vi "PicoScope3000aExampleEts.vi"() -> ()   [LabVIEW 2010]
uses:
  shared/PicoBuffers.ctl
  shared/Buffer and Transfer Settings.ctl
  shared/Acquisition Settings.ctl
  PicoScope3000aLib/PicoScope3000aAnalogChannelSettings.ctl
panel:
  out "Properties Panel":T1 {"Max Total Capture Time Available (sec)" format="%.3p"; "Sample Frequency" format="%.3p"; "Sample Rate" format="%.3p"; "Max Samples Available" format="%.3p"; "Total Capture Time (sec)" format="%.3p"}
  out "EtsTimeValues":i64[](array[numeric])
  in  "etsInterleave":i16=40
  in  "etsCycles":i16=200
  out "Max etsInterleave":i16
  out "Max etsCycles":i16
  in  "Trigger Settings":T2={"Trigger Enabled"=TRUE, "Trigger Source"=enum."Channel A", "Trigger Threshold (volts)"=0.0, "Trigger Direction"=2, "Trigger Delay (samples)"=0, "Auto Trigger Time (ms)"=1000} {"Trigger Direction" items=["Above", "Below", "Rising", "Falling", "Rising or Falling"]}
  in  "ETS Mode":u32(ring)=1 items=["PS3000A_ETS_OFF", "PS3000A_ETS_FAST", "PS3000A_ETS_SLOW"]
  in  "Channel A Settings":T3={"Enabled"=TRUE, "Coupling"=1, "Range"=6, "Analogue Offset"=0.0, "Bandwidth Limit"=0} {"Bandwidth Limit" items=["Full", "20MHz"]; "Range" items=["10 mV", "20 mV", "50 mV", "100 mV", "200 mV", "500 mV", "1 V", "2 V", "5 V", "10 V", "20 V", "50 V ", "100 V"]; "Coupling" items=["AC", "DC"]}
  out "overflow":i16 format="%010b"
  in  "Apply Settings":bool
  out "USB 3.0 device on non-USB 3.0 Port":bool=TRUE
  out "USB Powered":bool=TRUE
  out "Device Info":T4={"Driver Version"="0", "USB Version"="0", "Hardware"="0", "Variant"="0", "Batch and Serial"="0", "Cal Date"="0", "Kernel Version"="0", "Digital HW Version"="0", "Analogue HW Version"="0", "MSO"=FALSE, "Number of channels"=0}
  out "error out":errorcluster
  in  "Data file":path=path "PicoScope3000aExampleETS ChA Data"
  in  "Buffer and Transfer Settings":T5={"startIndex"=0, "Samples"=1000, "Down Sample Ratio"=1, "Down-Sample Mode"=0} {"Down-Sample Mode" items=["RAW none"=2147483648, "None"=0, "Aggregate"=1, "Decimate"=2, "Average"=4]; "Down Sample Ratio" step=1; "Samples" format="%_6p"}
  in  "Acquisition Settings":T6={"preTriggerSamples"=0, "postTriggerSamples"=1000, "timebase"=0} {"postTriggerSamples" format="%_6p"; "preTriggerSamples" format="%_6p"}
  in  "stop":bool
  out "Channel A":cluster{i32, sgl, "Data":dbl[]}(graph)
  in  "Serial Number":string
  in  "Use Serial Number":bool
  in  "error in (no error)":errorcluster
  # "Bit 0 = ChA"
  # "ETS mode on channel A only"
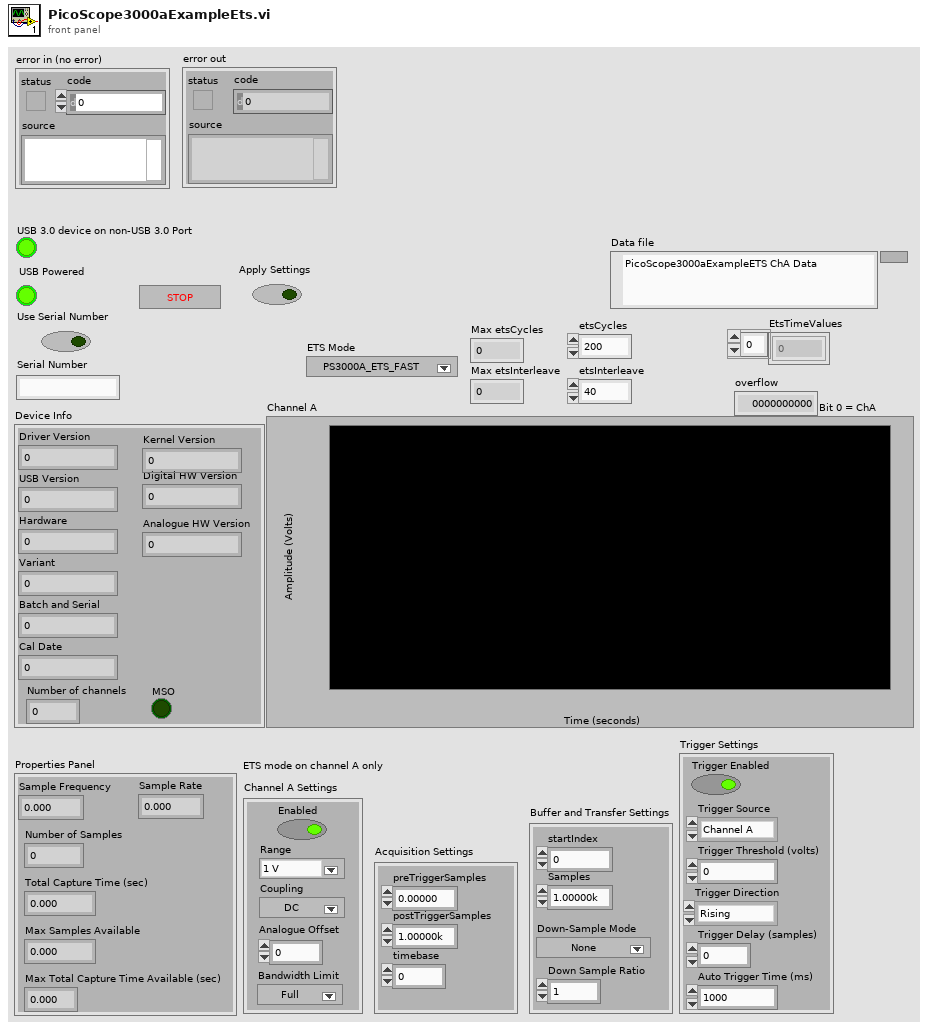
[diagram p1: front panel]
types:
  T1 = cluster{"Sample Frequency":sgl, "Sample Rate":sgl, "Max Samples Available":i32, "Number of Samples":u32, "Total Capture Time (sec) ":sgl, "Max Total Capture Time Available (sec)":sgl}
  T2 = cluster{"Trigger Enabled":bool, "Trigger Source":enum32{"Channel A", "Channel B", "Channel C", "Channel D", "Ext."}, "Trigger Threshold (volts)":dbl, "Trigger Direction":u32, "Trigger Delay (samples)":u32, "Auto Trigger Time (ms)":i16}
  T3 = typedef "PicoScope3000aAnalogChannelSettings.ctl" = cluster{"Enabled":bool, "Coupling":u32, "Range":u32, "Analogue Offset":sgl, "Bandwidth Limit":u32}
  T4 = cluster{"Driver Version":string, "USB Version":string, "Hardware":string, "Variant":string, "Batch and Serial":string, "Cal Date":string, "Kernel Version":string, "Digital HW Version":string, "Analogue HW Version":string, "MSO":bool, "Number of channels":i16}
  T5 = typedef "Buffer and Transfer Settings.ctl" = cluster{"startIndex":u64, "Samples":u64, "Down Sample Ratio":u64, "Down-Sample Mode":u32}
  T6 = typedef "Acquisition Settings.ctl" = cluster{"preTriggerSamples":u64, "postTriggerSamples":u64, "timebase":u32}
  T7 = typedef "PicoBuffers.ctl" = cluster{"Max Buffer Pointers":u64[][][], "Min Buffer Pointers":u64[][][], "StreamingDataInfo":cluster{"Channel":u32, "Down-Sample Mode":u32, "PICO_DATA_TYPE":enum32{"PICO_INT8_T", "PICO_INT16_T", "PICO_INT32_T", "PICO_UINT32_T", "PICO_INT64_T", ""}, "Samples":i32, "bufferIndex":u64, "startIndex":i32, "overflow":i16}[][]}
  T8 = enum16{"open", "open or create", "create or replace", "create", "open (read-only)"}
  T9 = cluster{"Channel A Buffer":i16[], "Channel B Buffer":i16[], "Channel C Buffer":i16[], "Channel D Buffer":i16[], "Channel E Buffer":i16[], "Channel F Buffer":i16[], "Channel G Buffer":i16[], "Channel H Buffer":i16[], "Port 0 Buffer":i16[], "Port 1 Buffer":i16[]}[]
  T10 = cluster{"Channel A Buffer":i16[], "Channel B Buffer":i16[], "Channel C Buffer":i16[], "Channel D Buffer":i16[], "Channel E Buffer":i16[], "Channel F Buffer":i16[], "Channel G Buffer":i16[], "Channel H Buffer":i16[], "Port 0 Buffer":i16[], "Port 1 Buffer":i16[]}
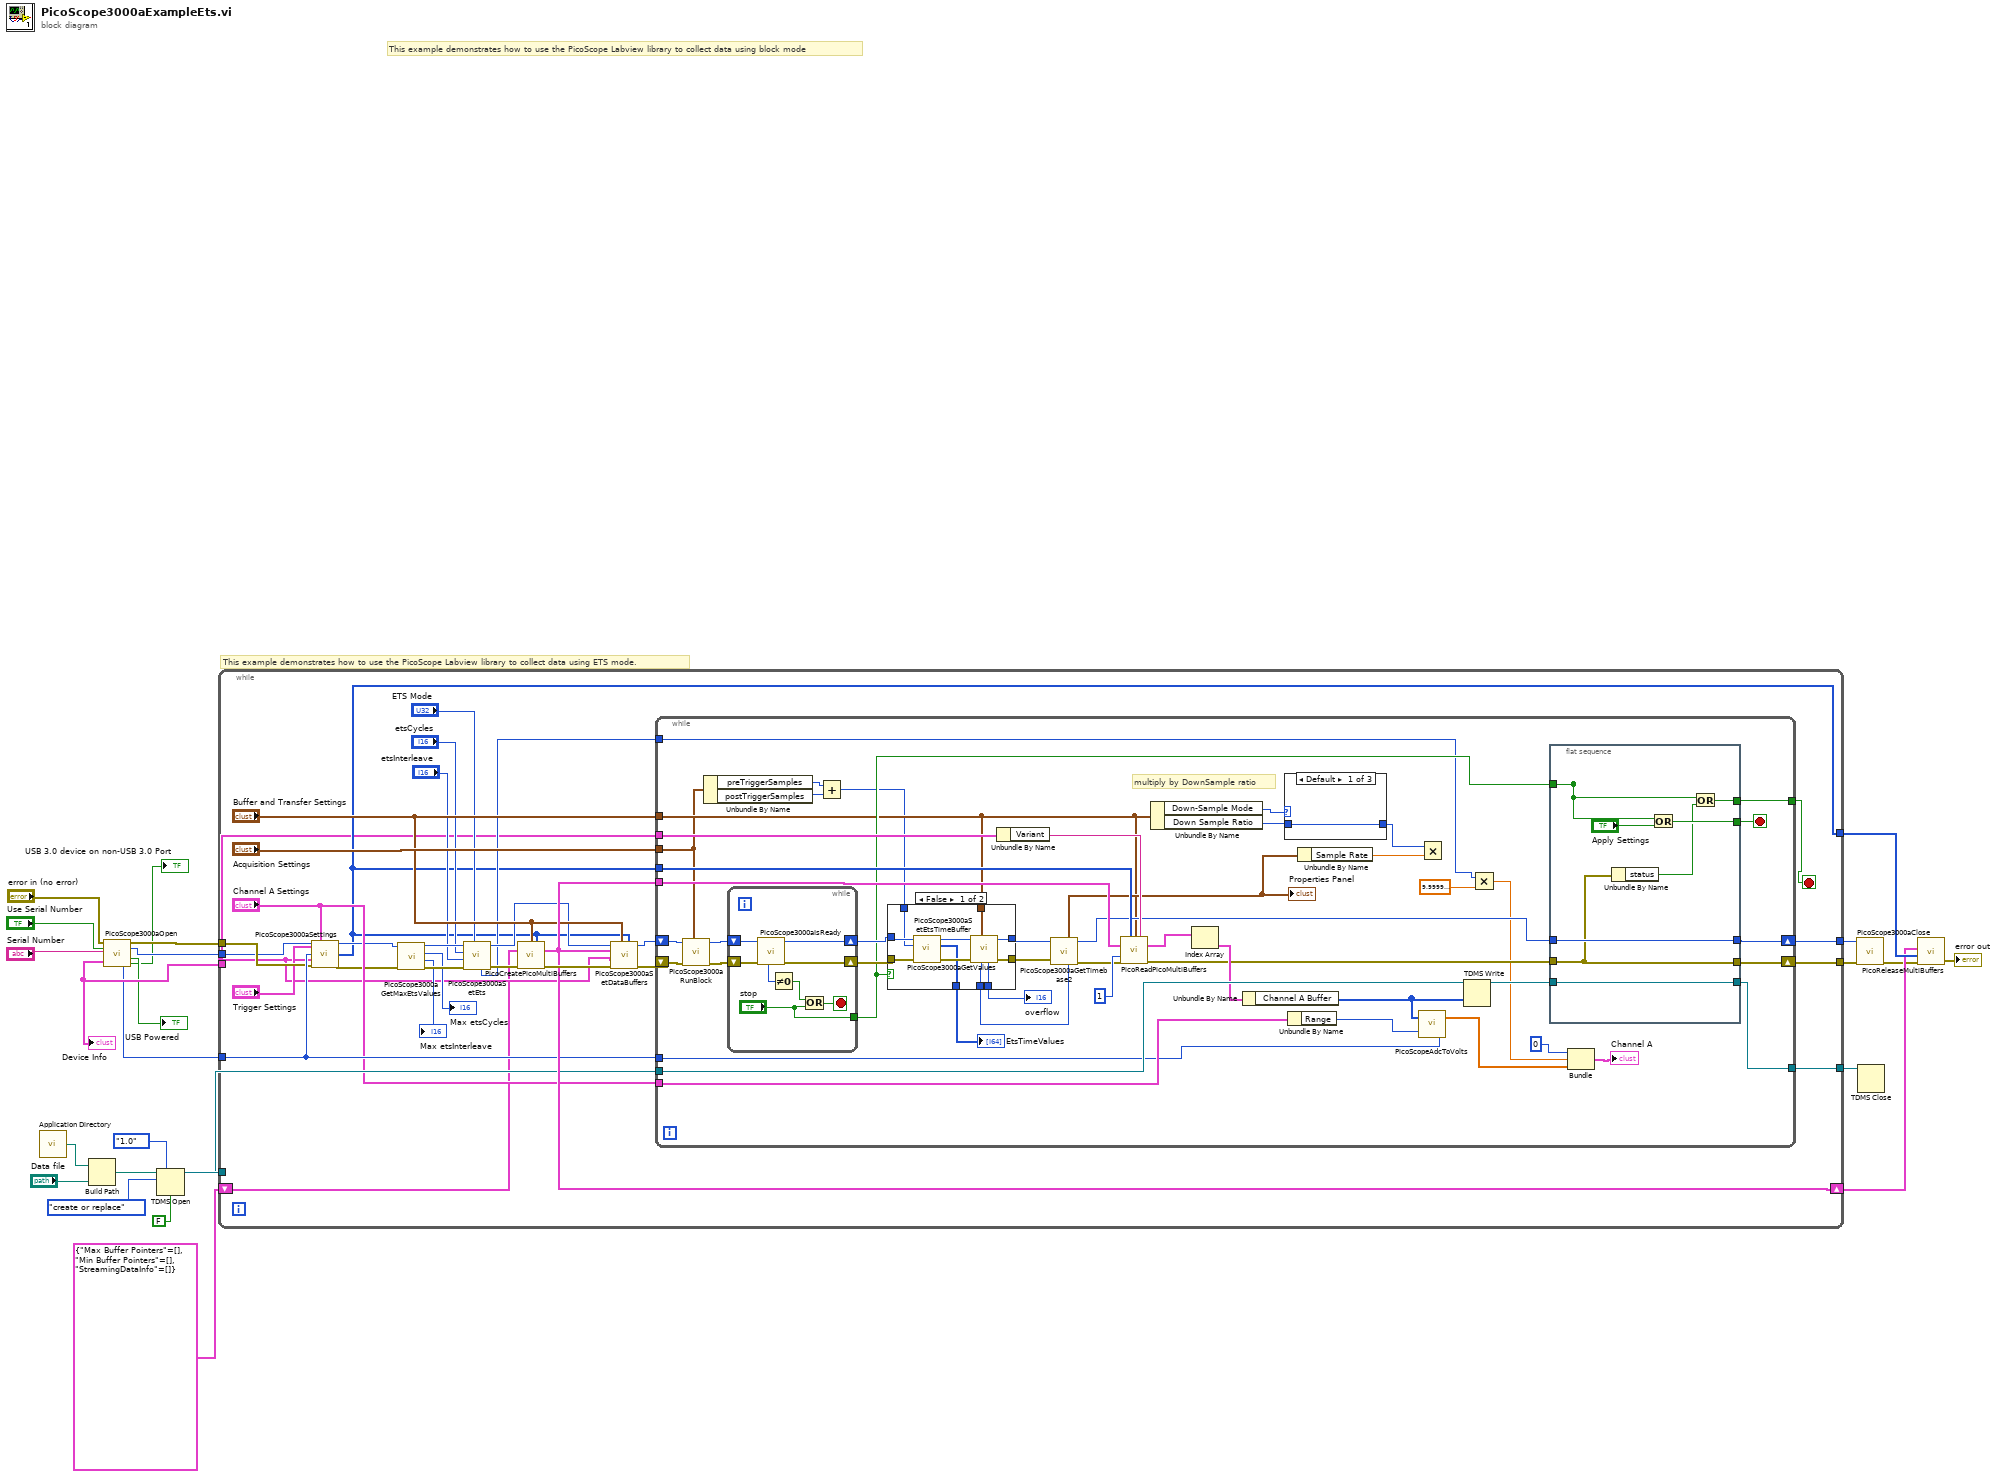
[diagram p0: block diagram]
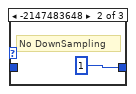
[diagram p3: hidden frame]
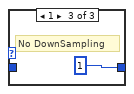
[diagram p4: hidden frame]
diagram:
  # "This example demonstrates how to use the PicoScope Labview library to collect data using ETS mode."
  # "This example demonstrates how to use the PicoScope Labview library to collect data using block mode"
  n1 = call <vilib>:"Application Directory.vi"() -> ("Application Directory"=w16:path)
  n2 = Build Path(base path=w16, name or relative path="Data file") -> (appended path=w17:path)
  n3 = call "PicoScope3000aOpen.vi"("error in (no error)"="error in (no error)", "Serial Number"="Serial Number", "Use Serial number"="Use Serial Number") -> ("error out"=w7:errorcluster, "handle"=w24:i16, "USB Powered"=→"USB Powered":bool, "Device Info"=w9:T4, "Max ADC value"=w5:i16, "USB 3.0 device on non-USB 3.0 Port"=→"USB 3.0 device on non-USB 3.0 Port":bool)  [unwired: 6 in, 1 out]
  "Device Info" <- w9
  n4 = TDMS Open(6:FALSE ("disable buffering? (T)"), 7:enum16{"1.0", "2.0"}."1.0" ("file format version (2.0)"), 10:T8."create or replace" ("operation (0:open)"), 11:w17) -> (3:w14:refnum<k34>)  [unwired: 2 in, 1 out]
  n5 = while {
    tunnel: w24 -> [w30]
    tunnel: w5 -> [w44]
    tunnel: [w28] -> w23
    tunnel: [w50] -> w15
    tunnel: w14 -> [w53]
    tunnel: w9 -> [w26]
    tunnel: w7 -> [w31]
    tunnel: [w51] -> w3
    tunnel: [w48] -> w6
    shift-right: [w54] -> w22
    shift-left: T7 {"Max Buffer Pointers"=[], "Min Buffer Pointers"=[], "StreamingDataInfo"=[]} ("Data Pointers") -> [w25]
    stop <- w49 stop-if-true
    n6 = call "PicoScope3000aSettings.vi"("handle in"=w30, "Channel A Settings"="Channel A Settings", "Trigger Settings"="Trigger Settings", "Max_adc"=w44, "Device Info"=w26, "error in"=w31) -> ("handle out"=w29:i16, "Enabled Array"=w28:i16[], "error out"=w32:errorcluster)  [unwired: 7 in]
    n7 = call "PicoScope3000aGetMaxEtsValues.vi"("error in (no error)"=w32, "handle in"=w29) -> ("error out"=w42:errorcluster, "Max etsInterleave"=→"Max etsInterleave":i16, "Max etsCycles"=→"Max etsCycles":i16, "handle out"=w39:i16)  [unwired: 6 in]
    n8 = call "PicoScope3000aSetEts.vi"("ETS Mode"="ETS Mode", "error in (no error)"=w42, "etsInterleave"="etsInterleave", "etsCycles"="etsCycles", "handle in"=w39) -> ("error out"=w41:errorcluster, "handle out"=w40:i16, "sampleTimePicoseconds"=w38:i32)  [unwired: 4 in]
    n9 = call "PicoCreatePicoMultiBuffers.vi"("Buffer and Transfer Settings"="Buffer and Transfer Settings", "enabled array"=w28, "Data Pointers In"=w25, "error in (no error)"=w41) -> ("Data Pointers"=w54:T7, "error out"=w55:errorcluster)  [unwired: 10 in]
    n10 = call "PicoScope3000aSetDataBuffers.vi"("enabled array"=w28, "Buffer and Transfer Settings"="Buffer and Transfer Settings", "error in (no error)"=w55, "Device Info"=w26, "Data Pointers In"=w54, "handle in"=w40) -> ("error out"=w47:errorcluster, "handle out"=w46:i16)  [unwired: 4 in]
    n11 = while {
      tunnel: w54 -> [w104]
      tunnel: "Buffer and Transfer Settings" -> [w66]
      tunnel: w28 -> [w96]
      tunnel: "Channel A Settings" -> [w95]
      tunnel: "Acquisition Settings" -> [w59]
      tunnel: w44 -> [w94]
      tunnel: w26 -> [w91]
      tunnel: [w81] -> w49
      shift-right: [w85] -> w51
      shift-left: w47 -> [w75]
      shift-right: [w79] -> w48
      shift-left: w46 -> [w76]
      tunnel: w53 -> [w103]
      tunnel: [w83] -> w50
      tunnel: w38 -> [w63]
      stop <- w80 stop-if-true
      # "multiply by DownSample ratio"
      n12 = call "PicoScope3000aRunBlock.vi"("Acquisition Settings"=w59, "error in (no error)"=w75, "handle in"=w76) -> ("error out"=w98:errorcluster, "handle out"=w97:i16)  [unwired: 5 in, 2 out]
      n13 = Unbundle By Name(w59) -> ("preTriggerSamples"=w58:u64, "postTriggerSamples"=w57:u64)
      n14 = while {
        shift-right: [w132] -> w77
        shift-left: w98 -> [w133]
        shift-right: [w131] -> w78
        shift-left: w97 -> [w130]
        tunnel: ["stop"] -> w74
        stop <- w127 stop-if-true
        n15 = call "PicoScope3000aIsReady.vi"("error in (no error)"=w133, "handle in"=w130) -> ("error out"=w132:errorcluster, "handle out"=w131:i16, "ready"=w129:i16)  [unwired: 7 in]
        n16 = Not Equal To 0?(x=w129) -> (x != 0?=w128:bool)
        n17 = Or(x=w128, y="stop") -> (x .or. y?=w127:bool)
      }
      n18 = Add(x=w58, y=w57) -> (x+y=w56:u64)
      n19 = case shown="False" w74 {
        tunnel: w77 -> [w110 w116]
        tunnel: w78 -> [w107 w117]
        tunnel: [w115 w117] -> w69
        tunnel: [w114 w116] -> w70
        tunnel: w66 -> [w113 _]
        tunnel: [w112 _] -> w73
        tunnel: [w111 _] -> w72
        tunnel: [w106 _] -> w62
        tunnel: w56 -> [w105 _]
        frame False {
          n20 = call "PicoScope3000aSetEtsTimeBuffer.vi"("error in (no error)"=w110, "bufferLth"=w105, "handle in"=w107) -> ("error out"=w109:errorcluster, "EtsTimeValues"=w106:i64[], "handle out"=w108:i16)  [unwired: 6 in]
          n21 = call "PicoScope3000aGetValues.vi"("Buffer and Transfer Settings"=w113, "error in (no error)"=w109, "handle in"=w108) -> ("error out"=w114:errorcluster, "handle out"=w115:i16, "overflow"=w112:i16, "noOfSamples"=w111:u64)  [unwired: 5 in]
        }
        frame True {
        }
      }
      "overflow" <- w73
      "EtsTimeValues" <- w62
      n22 = Unbundle By Name(w91) -> ("Variant"=w92:string)
      n23 = call "PicoScope3000aGetTimebase2.vi"("Number of Samples"=w72, "error in (no error)"=w70, "handle in"=w69) -> ("error out"=w68:errorcluster, "handle out"=w67:i16, "Properties Panel"=w71:T1)  [unwired: 6 in]
      "Properties Panel" <- w71
      n24 = call "PicoReadPicoMultiBuffers.vi"("enabled array"=w96, "Buffer and Transfer Settings"=w66, "Variant"=w92, "Data Pointers"=w104, "No of Buffers"=1, "error in (no error)"=w68) -> ("MultiBuffers (Max or non-aggregated)"=w102:T9, "error out"=w82:errorcluster)  [unwired: 7 in, 1 out]
      n25 = Unbundle By Name(w66) -> ("Down-Sample Mode"=w100:u32, "Down Sample Ratio"=w101:u64)
      n26 = Index Array(array=w102) -> (element=w86:T10)  [unwired: 1 in]
      n27 = Unbundle By Name(w86) -> ("Channel A Buffer"=w87:i16[])
      n28 = case shown="Default" w100 {
        tunnel: [w134 u64 1 ("Down Sample Ratio") u64 1 ("Down Sample Ratio")] -> w99
        tunnel: w101 -> [w134 _ _]
        frame Default {
        }
        frame -2147483648 {
          # "No DownSampling"
        }
        frame 1 {
          # "No DownSampling"
        }
      }
      n29 = Unbundle By Name(w95) -> ("Range"=w88:u32)
      n30 = Unbundle By Name(w71) -> ("Sample Rate"=w93:sgl)
      n31 = call "PicoScopeAdcToVolts.vi"("Max_adc"=w94, "Range Index"=w88, "Data"=w87) -> ("Data"=w61:dbl[])
      n32 = Multiply(x=w99, y=w93) -> ()  [unwired: 1 out]
      n33 = TDMS Write(0:w103, 9:w87) -> (4:w84:refnum<k34>)  [unwired: 4 in, 3 out]
      n34 = Multiply(x=w63, y=sgl 1e-12) -> (x*y=w64:sgl)
      n35 = flat-sequence {
        tunnel: [w125] -> w80
        tunnel: [w118] -> _
        tunnel: [w122] -> w81
        tunnel: w67 -> [w121]
        tunnel: [w121] -> w79
        tunnel: w82 -> [w120]
        tunnel: [w120] -> w85
        tunnel: [w119] -> w83
        tunnel: w84 -> [w119]
        tunnel: w74 -> [w118]
        frame #0 {
          n36 = Unbundle By Name(w120) -> ("status"=w123:bool)
          n37 = Or(x=w118, y="Apply Settings") -> (x .or. y?=w125:bool)
          n38 = Or(x=w118, y=w123) -> (x .or. y?=w122:bool)
        }
      }
      n39 = Bundle(0, w64, "Data"=w61) -> (→"Channel A":cluster{i32, sgl, "Data":dbl[]})  [unwired: 1 in]
    }
  }
  n40 = call "PicoScope3000aClose.vi"("error in (no error)"=w3, "handle in"=w6) -> ("error out"=w2:errorcluster)  [unwired: 8 in, 1 out]
  n41 = TDMS Close(11:w15) -> ()  [unwired: 1 in, 2 out]
  n42 = call "PicoReleaseMultiBuffers.vi"("error in (no error)"=w2, "Enabled array"=w23, "Data Pointers"=w22) -> ("error out"=→"error out":errorcluster)  [unwired: 7 in, 1 out]
